vi "Control.vi"() -> ()   [LabVIEW 2023, in "BigSkyControl.lvlib"]
uses:
  BigSkyControl.lvlib
  VISAGlobal.vi
panel:
  out "Temperature(C)":dbl=40.0
  in  "Flashlamp mode":bool
  out "Response History":string="Voltage m0725 V\r\ntemp. CG 40 d  \r\nfire ext       \r\n\rtemp. CG 40 d  \r\nfire ext       \rtemp. CG 40 d  \r\nVoltage m0725 V\r\nLP synch :  1  \r\nstandby        \r\n"
  in  "Command (no > or \\r\\n)":string
  in  "Send Command":bool
  in  "Frequency[Hz]":dbl=10.0 min=0.01 max=56.0 step=0.01 format="%.2g"
  in  "Query Frequency":bool
  in  "Set Frequency":bool
  in  "Query Shutter":bool
  in  "Single QSwitch":bool
  in  "Stop QSwitch":bool
  in  "Start QSwitch":bool
  in  "Query Voltage":bool
  in  "Set Voltage":bool
  in  "Stop":bool
  out "Voltage Reported":dbl=725.0 format="%_4f"
  in  "Voltage[V]":dbl(slide)=725.0 min=700.0 max=950.0 step=5.0 scale=700.0..950.0
  in  "Stop Lamps":bool
  in  "Warmup Lamps":bool
  out "Response":string="Voltage m0725 V\r\n"
  in  "Close shutter":bool
  in  "Open shutter":bool
  in  "VISA resource name":refnum<visa-resource-name>="COM16"
  # "BigSky Laser Control Panel"
  # "System"
  # "Lamp Control"
  # "Q-Switch Control - WILL FIRE LASER"
  # "Shutter Control"
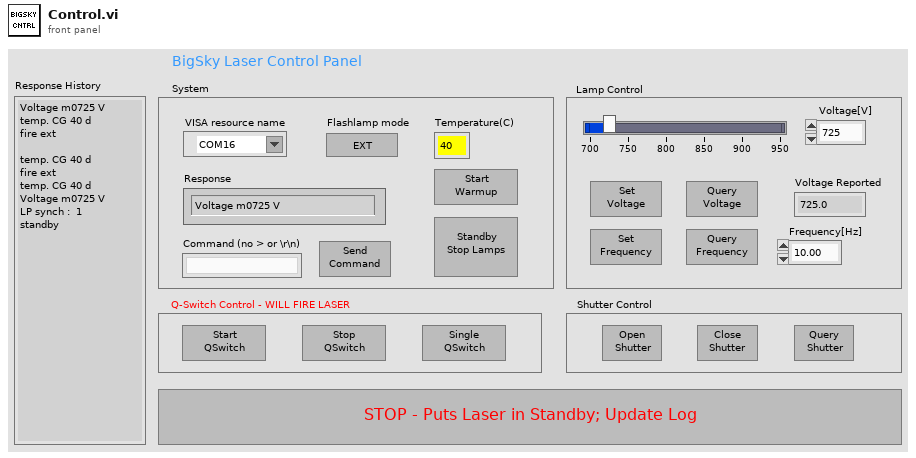
[diagram p1: front panel]
types:
  T1 = enum8{"Enabled", "Disabled", "Disabled and Grayed Out"}
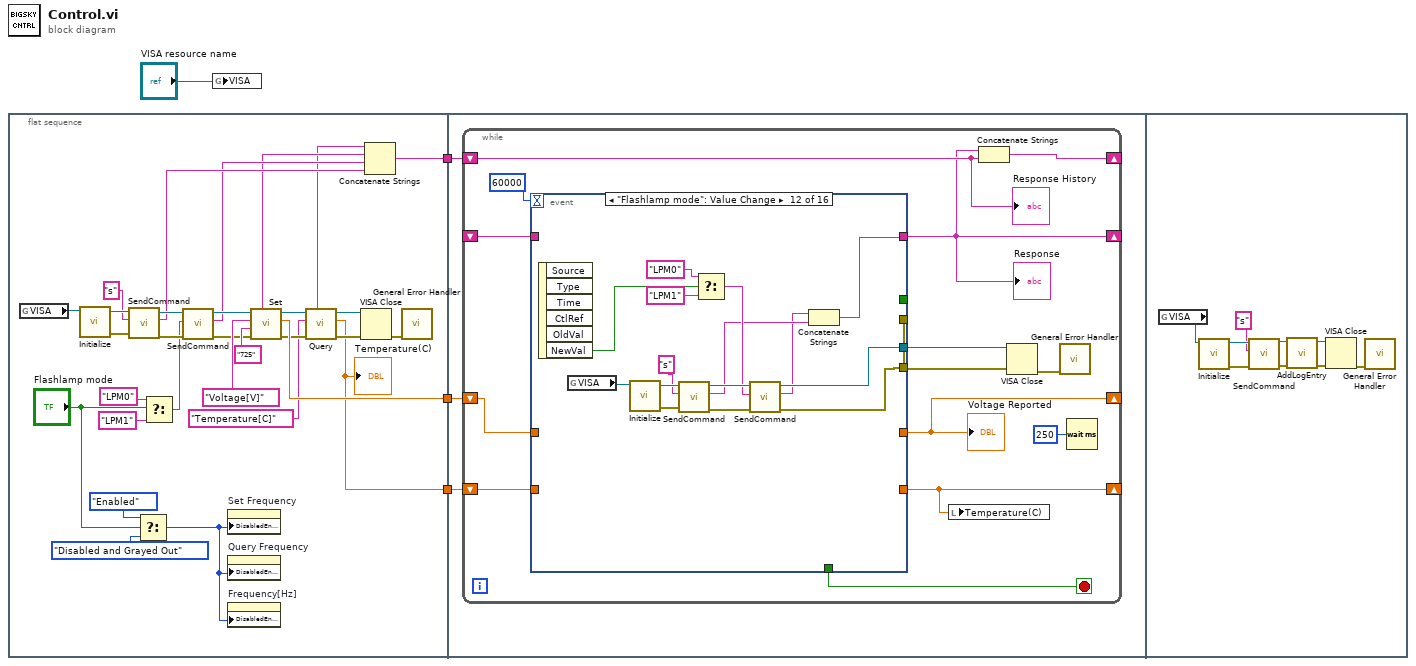
[diagram p0: block diagram]
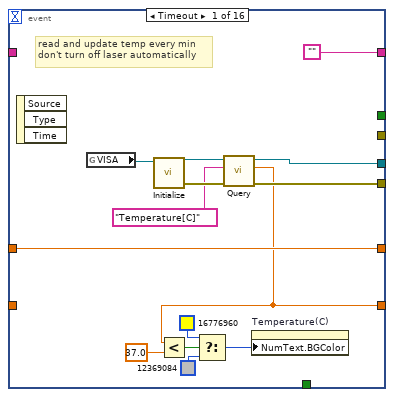
[diagram p2: hidden frame]
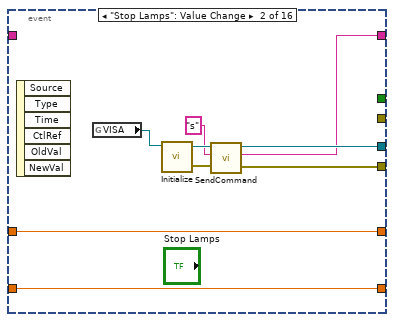
[diagram p3: hidden frame]
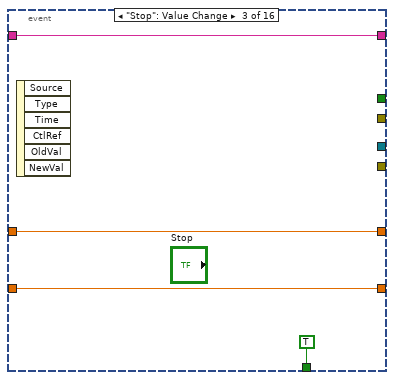
[diagram p4: hidden frame]
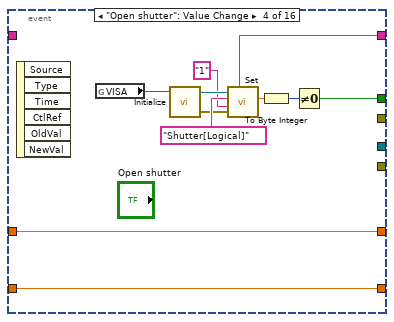
[diagram p5: hidden frame]
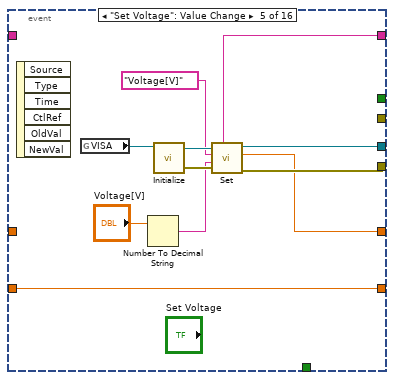
[diagram p6: hidden frame]
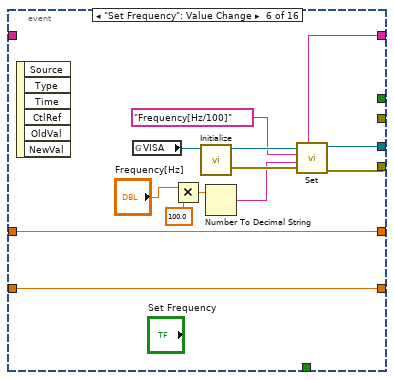
[diagram p7: hidden frame]
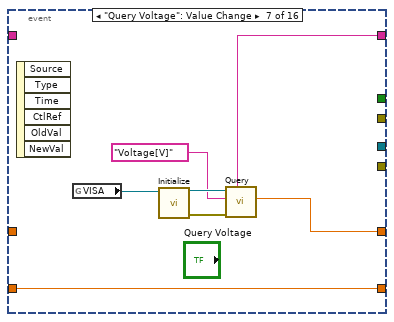
[diagram p8: hidden frame]
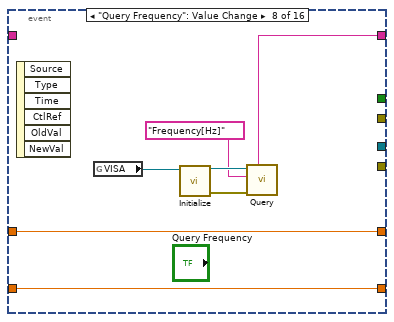
[diagram p9: hidden frame]
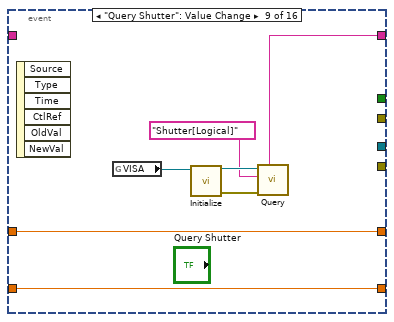
[diagram p10: hidden frame]
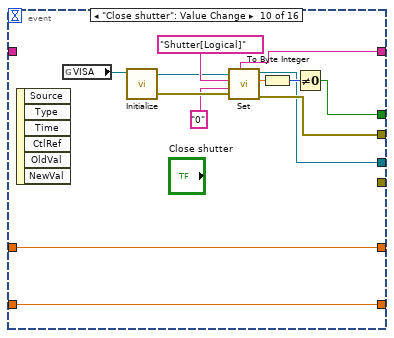
[diagram p11: hidden frame]
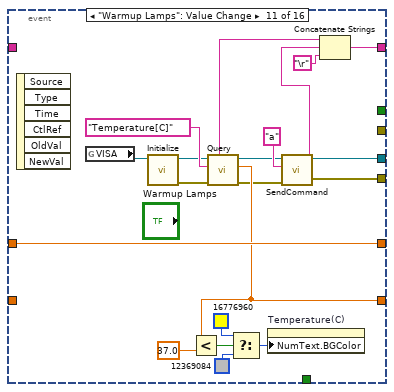
[diagram p12: hidden frame]
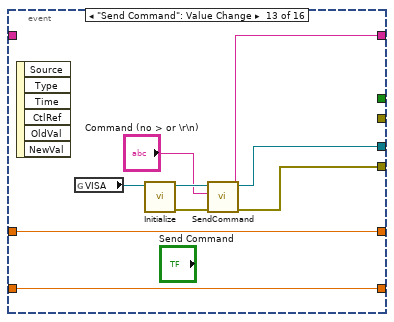
[diagram p13: hidden frame]
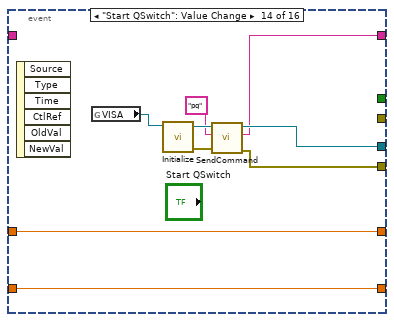
[diagram p14: hidden frame]
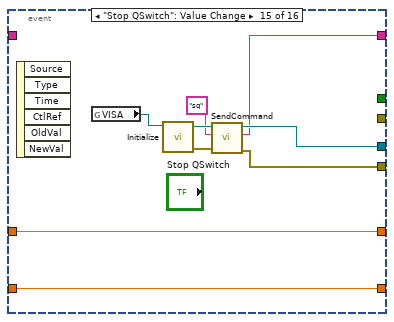
[diagram p15: hidden frame]
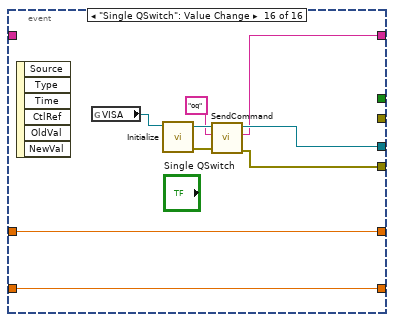
[diagram p16: hidden frame]
diagram:
  n1 = flat-sequence {
    tunnel: [w27] -> w3
    tunnel: [w20] -> w2
    tunnel: [w5] -> w1
    tunnel: w3 -> [w37]
    tunnel: w2 -> [w36]
    tunnel: w1 -> [w35]
    frame #0 {
      n2 = global read "VISAGlobal.vi" "VISA"() -> (w31:refnum<visa-resource-name>)
      n3 = call "Initialize.vi"("VISA resource name"=w31) -> ("error out"=w33:errorcluster, "VISA resource name out"=w34:refnum<visa-resource-name>)  [unwired: 7 in]
      n4 = call "SendCommand.vi"("error"=w33, "write buffer (don't include >\\r\\n)"="s" ("write buffer (don't include >\\r\\n)"), "VISA resource name"=w34) -> ("error out"=w24:errorcluster, "Response"=w9:string, "VISA resource name out"=w26:refnum<visa-resource-name>)  [unwired: 6 in]
      n5 = Select(t=T1."Enabled" ("Disabled"), s="Flashlamp mode", f=T1."Disabled and Grayed Out" ("Disabled")) -> (s? t:f=w10:T1)
      n6 = Select(t="LPM0" ("write buffer (don't include >\\r\\n)"), s="Flashlamp mode", f="LPM1" ("write buffer (don't include >\\r\\n)")) -> (s? t:f=w22:string)
      n7 = call "SendCommand.vi"("error"=w24, "write buffer (don't include >\\r\\n)"=w22, "VISA resource name"=w26) -> ("error out"=w23:errorcluster, "Response"=w8:string, "VISA resource name out"=w25:refnum<visa-resource-name>)  [unwired: 6 in]
      n8 = property on="Set Frequency" class="Bool"("DisabledEnum"=w10) -> ()  [unwired: 2 in, 2 out]
      n9 = property on="Query Frequency" class="Bool"("DisabledEnum"=w10) -> ()  [unwired: 2 in, 2 out]
      n10 = property on="Frequency[Hz]" class="DigNum (strict)"("DisabledEnum"=w10) -> ()  [unwired: 2 in, 2 out]
      n11 = call "Set.vi"("error"=w23, "Input Command String"="725", "Quantity"="Voltage[V]", "VISA resource name"=w25) -> ("error out"=w17:errorcluster, "Returned"=w20:dbl, "VISA resource name out"=w19:refnum<visa-resource-name>, "Response"=w7:string)  [unwired: 2 in]
      n12 = call "Query.vi"("error"=w17, "Quantity"="Temperature[C]", "VISA resource name"=w19) -> ("error out"=w16:errorcluster, "Value"=w5:dbl, "VISA resource name out"=w18:refnum<visa-resource-name>, "Response"=w6:string)  [unwired: 3 in]
      "Temperature(C)" <- w5
      n13 = VISA Close(VISA resource name=w18, error in (no error)=w16) -> (error out=w30:errorcluster)
      n14 = Concatenate Strings(w6, w7, w8, w9) -> (w27:string)
      n15 = call <vilib>:"General Error Handler.vi"("error in (no error)"=w30) -> ()  [unwired: 10 in, 5 out]
    }
    frame #1 {
      n16 = while {
        shift-right: [w40] -> _
        shift-left: _ -> [w45]
        shift-right: [w44] -> _
        shift-left: w36 -> [w43]
        shift-right: [w42] -> _
        shift-left: w37 -> [w41]
        shift-right: [w38] -> _
        shift-left: w35 -> [w39]
        stop <- w47 stop-if-true
        n17 = event shown="[11] \"Flashlamp mode\": Value Change" {
          selector: _ -> [_ _ _ _ _ _ _ _ _ _ _ _ _ _ _ _]
          dyn-events: _ -> [_ _ _ _ _ _ _ _ _ _ _ _ _ _ _ _]
          timeout: 60000 -> [_ _ _ _ _ _ _ _ _ _ _ _ _ _ _ _]
          tunnel: ["" w68 w77 w86 w97 w110 w115 w123 w130 w144 w157 w172 w186 w194 w203 w212] -> w40
          tunnel: [_ _ _ w83 _ _ _ _ _ w141 _ _ _ _ _ _] -> _
          tunnel: [_ _ _ _ _ _ _ _ _ w139 _ _ _ _ _ _] -> w51
          tunnel: [w64 w70 _ _ w93 w108 _ _ _ w138 w151 w171 w188 w195 w204 w213] -> w50
          tunnel: [w63 w69 _ _ w92 w107 _ _ _ _ w148 w170 w187 w196 w205 w214] -> _
          tunnel: [_ _ TRUE _ _ _ _ _ _ _ _ _ _ _ _ _] -> w47
          tunnel: [w65 w67 w76 w80 w91 w101 w116 w122 w129 w136 w165 _ w185 w192 w202 w211] -> w44
          tunnel: w45 -> [_ _ w77 _ _ _ _ _ _ _ _ _ _ _ _ _]
          tunnel: w43 -> [w65 w67 w76 w80 _ w101 _ w122 w129 w136 w165 _ w185 w192 w202 w211]
          tunnel: w39 -> [_ w66 w75 w79 w90 w102 w114 w121 w128 w135 _ _ w183 w193 w201 w210]
          tunnel: [w58 w66 w75 w79 w90 w102 w114 w121 w128 w135 w162 _ w183 w193 w201 w210] -> w38
          event Timeout {
            # "read and update temp every min\ndon't turn off laser automatically"
            n18 = event-data() -> ()  [unwired: 1 in, 3 out]
            n19 = global read "VISAGlobal.vi" "VISA"() -> (w60:refnum<visa-resource-name>)
            n20 = call "Initialize.vi"("VISA resource name"=w60) -> ("error out"=w61:errorcluster, "VISA resource name out"=w62:refnum<visa-resource-name>)  [unwired: 7 in]
            n21 = call "Query.vi"("error"=w61, "Quantity"="Temperature[C]", "VISA resource name"=w62) -> ("error out"=w63:errorcluster, "Value"=w58:dbl, "VISA resource name out"=w64:refnum<visa-resource-name>)  [unwired: 3 in, 1 out]
            n22 = Less?(x=w58, y=37.0) -> (x < y?=w54:bool)
            n23 = Select(t=u32 16776960 ("Color"), s=w54, f=u32 12369084 ("Color")) -> (s? t:f=w53:u32)
            n24 = property on="Temperature(C)" class="DigNum (strict)"("NumText.BGColor"=w53) -> ()  [unwired: 2 in, 2 out]
          }
          event "Stop Lamps": Value Change {
            n25 = event-data() -> ()  [unwired: 1 in, 6 out]
            n26 = global read "VISAGlobal.vi" "VISA"() -> (w71:refnum<visa-resource-name>)
            n27 = call "Initialize.vi"("VISA resource name"=w71) -> ("error out"=w73:errorcluster, "VISA resource name out"=w74:refnum<visa-resource-name>)  [unwired: 7 in]
            n28 = call "SendCommand.vi"("error"=w73, "write buffer (don't include >\\r\\n)"="s" ("write buffer (don't include >\\r\\n)"), "VISA resource name"=w74) -> ("error out"=w69:errorcluster, "Response"=w68:string, "VISA resource name out"=w70:refnum<visa-resource-name>)  [unwired: 6 in]
          }
          event "Stop": Value Change {
            n29 = event-data() -> ()  [unwired: 1 in, 6 out]
          }
          event "Open shutter": Value Change {
            n30 = event-data() -> ()  [unwired: 1 in, 6 out]
            n31 = global read "VISAGlobal.vi" "VISA"() -> (w81:refnum<visa-resource-name>)
            n32 = call "Initialize.vi"("VISA resource name"=w81) -> ("error out"=w87:errorcluster, "VISA resource name out"=w88:refnum<visa-resource-name>)  [unwired: 7 in]
            n33 = call "Set.vi"("error"=w87, "Input Command String"="1", "Quantity"="Shutter[Logical]", "VISA resource name"=w88) -> ("Returned"=w85:dbl, "Response"=w86:string)  [unwired: 2 in, 2 out]
            n34 = To Byte Integer(number=w85) -> (8bit integer=w84:i8)
            n35 = Not Equal To 0?(x=w84) -> (x != 0?=w83:bool)
          }
          event "Set Voltage": Value Change {
            n36 = event-data() -> ()  [unwired: 1 in, 6 out]
            n37 = global read "VISAGlobal.vi" "VISA"() -> (w98:refnum<visa-resource-name>)
            n38 = Number To Decimal String(number="Voltage[V]") -> (decimal integer string=w94:string)  [unwired: 1 in]
            n39 = call "Initialize.vi"("VISA resource name"=w98) -> ("error out"=w99:errorcluster, "VISA resource name out"=w100:refnum<visa-resource-name>)  [unwired: 7 in]
            n40 = call "Set.vi"("error"=w99, "Input Command String"=w94, "Quantity"="Voltage[V]", "VISA resource name"=w100) -> ("error out"=w92:errorcluster, "Returned"=w91:dbl, "VISA resource name out"=w93:refnum<visa-resource-name>, "Response"=w97:string)  [unwired: 2 in]
          }
          event "Set Frequency": Value Change {
            n41 = event-data() -> ()  [unwired: 1 in, 6 out]
            n42 = global read "VISAGlobal.vi" "VISA"() -> (w111:refnum<visa-resource-name>)
            n43 = Multiply(x="Frequency[Hz]", y=100.0) -> (x*y=w104:dbl)
            n44 = call "Initialize.vi"("VISA resource name"=w111) -> ("error out"=w112:errorcluster, "VISA resource name out"=w113:refnum<visa-resource-name>)  [unwired: 7 in]
            n45 = Number To Decimal String(number=w104) -> (decimal integer string=w109:string)  [unwired: 1 in]
            n46 = call "Set.vi"("error"=w112, "Input Command String"=w109, "Quantity"="Frequency[Hz/100]", "VISA resource name"=w113) -> ("error out"=w107:errorcluster, "VISA resource name out"=w108:refnum<visa-resource-name>, "Response"=w110:string)  [unwired: 2 in, 1 out]
          }
          event "Query Voltage": Value Change {
            n47 = event-data() -> ()  [unwired: 1 in, 6 out]
            n48 = global read "VISAGlobal.vi" "VISA"() -> (w118:refnum<visa-resource-name>)
            n49 = call "Initialize.vi"("VISA resource name"=w118) -> ("error out"=w119:errorcluster, "VISA resource name out"=w120:refnum<visa-resource-name>)  [unwired: 7 in]
            n50 = call "Query.vi"("error"=w119, "Quantity"="Voltage[V]", "VISA resource name"=w120) -> ("Value"=w116:dbl, "Response"=w115:string)  [unwired: 3 in, 2 out]
          }
          event "Query Frequency": Value Change {
            n51 = event-data() -> ()  [unwired: 1 in, 6 out]
            n52 = global read "VISAGlobal.vi" "VISA"() -> (w125:refnum<visa-resource-name>)
            n53 = call "Initialize.vi"("VISA resource name"=w125) -> ("error out"=w126:errorcluster, "VISA resource name out"=w127:refnum<visa-resource-name>)  [unwired: 7 in]
            n54 = call "Query.vi"("error"=w126, "Quantity"="Frequency[Hz]", "VISA resource name"=w127) -> ("Response"=w123:string)  [unwired: 3 in, 3 out]
          }
          event "Query Shutter": Value Change {
            n55 = event-data() -> ()  [unwired: 1 in, 6 out]
            n56 = global read "VISAGlobal.vi" "VISA"() -> (w132:refnum<visa-resource-name>)
            n57 = call "Initialize.vi"("VISA resource name"=w132) -> ("error out"=w133:errorcluster, "VISA resource name out"=w134:refnum<visa-resource-name>)  [unwired: 7 in]
            n58 = call "Query.vi"("error"=w133, "Quantity"="Shutter[Logical]", "VISA resource name"=w134) -> ("Response"=w130:string)  [unwired: 3 in, 3 out]
          }
          event "Close shutter": Value Change {
            n59 = event-data() -> ()  [unwired: 1 in, 6 out]
            n60 = global read "VISAGlobal.vi" "VISA"() -> (w137:refnum<visa-resource-name>)
            n61 = call "Initialize.vi"("VISA resource name"=w137) -> ("error out"=w145:errorcluster, "VISA resource name out"=w146:refnum<visa-resource-name>)  [unwired: 7 in]
            n62 = call "Set.vi"("error"=w145, "Input Command String"="0", "Quantity"="Shutter[Logical]", "VISA resource name"=w146) -> ("error out"=w139:errorcluster, "Returned"=w143:dbl, "VISA resource name out"=w138:refnum<visa-resource-name>, "Response"=w144:string)  [unwired: 2 in]
            n63 = To Byte Integer(number=w143) -> (8bit integer=w142:i8)
            n64 = Not Equal To 0?(x=w142) -> (x != 0?=w141:bool)
          }
          event "Warmup Lamps": Value Change {
            n65 = event-data() -> ()  [unwired: 1 in, 6 out]
            n66 = global read "VISAGlobal.vi" "VISA"() -> (w166:refnum<visa-resource-name>)
            n67 = call "Initialize.vi"("VISA resource name"=w166) -> ("error out"=w150:errorcluster, "VISA resource name out"=w153:refnum<visa-resource-name>)  [unwired: 7 in]
            n68 = call "Query.vi"("error"=w150, "Quantity"="Temperature[C]", "VISA resource name"=w153) -> ("error out"=w149:errorcluster, "Value"=w162:dbl, "VISA resource name out"=w152:refnum<visa-resource-name>, "Response"=w156:string)  [unwired: 3 in]
            n69 = Less?(x=w162, y=37.0) -> (x < y?=w161:bool)
            n70 = Select(t=u32 16776960 ("Color"), s=w161, f=u32 12369084 ("Color")) -> (s? t:f=w160:u32)
            n71 = property on="Temperature(C)" class="DigNum (strict)"("NumText.BGColor"=w160) -> ()  [unwired: 2 in, 2 out]
            n72 = call "SendCommand.vi"("error"=w149, "write buffer (don't include >\\r\\n)"="a" ("write buffer (don't include >\\r\\n)"), "VISA resource name"=w152) -> ("error out"=w148:errorcluster, "Response"=w155:string, "VISA resource name out"=w151:refnum<visa-resource-name>)  [unwired: 6 in]
            n73 = Concatenate Strings(w156, w155, "\r") -> (w157:string)
          }
          event "Flashlamp mode": Value Change {
            n74 = event-data() -> ("NewVal"=w174:bool)  [unwired: 1 in, 5 out]
            n75 = global read "VISAGlobal.vi" "VISA"() -> (w180:refnum<visa-resource-name>)
            n76 = call "Initialize.vi"("VISA resource name"=w180) -> ("error out"=w181:errorcluster, "VISA resource name out"=w182:refnum<visa-resource-name>)  [unwired: 7 in]
            n77 = call "SendCommand.vi"("error"=w181, "write buffer (don't include >\\r\\n)"="s" ("write buffer (don't include >\\r\\n)"), "VISA resource name"=w182) -> ("error out"=w178:errorcluster, "Response"=w169:string, "VISA resource name out"=w177:refnum<visa-resource-name>)  [unwired: 6 in]
            n78 = Select(t="LPM0" ("write buffer (don't include >\\r\\n)"), s=w174, f="LPM1" ("write buffer (don't include >\\r\\n)")) -> (s? t:f=w173:string)
            n79 = call "SendCommand.vi"("error"=w178, "write buffer (don't include >\\r\\n)"=w173, "VISA resource name"=w177) -> ("error out"=w170:errorcluster, "Response"=w168:string, "VISA resource name out"=w171:refnum<visa-resource-name>)  [unwired: 6 in]
            n80 = Concatenate Strings(w168, w169) -> (w172:string)
          }
          event "Send Command": Value Change {
            n81 = event-data() -> ()  [unwired: 1 in, 6 out]
            n82 = global read "VISAGlobal.vi" "VISA"() -> (w189:refnum<visa-resource-name>)
            n83 = call "Initialize.vi"("VISA resource name"=w189) -> ("error out"=w190:errorcluster, "VISA resource name out"=w191:refnum<visa-resource-name>)  [unwired: 7 in]
            n84 = call "SendCommand.vi"("error"=w190, "write buffer (don't include >\\r\\n)"="Command (no > or \\r\\n)", "VISA resource name"=w191) -> ("error out"=w187:errorcluster, "Response"=w186:string, "VISA resource name out"=w188:refnum<visa-resource-name>)  [unwired: 6 in]
          }
          event "Start QSwitch": Value Change {
            n85 = event-data() -> ()  [unwired: 1 in, 6 out]
            n86 = global read "VISAGlobal.vi" "VISA"() -> (w197:refnum<visa-resource-name>)
            n87 = call "Initialize.vi"("VISA resource name"=w197) -> ("error out"=w199:errorcluster, "VISA resource name out"=w200:refnum<visa-resource-name>)  [unwired: 7 in]
            n88 = call "SendCommand.vi"("error"=w199, "write buffer (don't include >\\r\\n)"="pq" ("write buffer (don't include >\\r\\n)"), "VISA resource name"=w200) -> ("error out"=w196:errorcluster, "Response"=w194:string, "VISA resource name out"=w195:refnum<visa-resource-name>)  [unwired: 6 in]
          }
          event "Stop QSwitch": Value Change {
            n89 = event-data() -> ()  [unwired: 1 in, 6 out]
            n90 = global read "VISAGlobal.vi" "VISA"() -> (w206:refnum<visa-resource-name>)
            n91 = call "Initialize.vi"("VISA resource name"=w206) -> ("error out"=w208:errorcluster, "VISA resource name out"=w209:refnum<visa-resource-name>)  [unwired: 7 in]
            n92 = call "SendCommand.vi"("error"=w208, "write buffer (don't include >\\r\\n)"="sq" ("write buffer (don't include >\\r\\n)"), "VISA resource name"=w209) -> ("error out"=w205:errorcluster, "Response"=w203:string, "VISA resource name out"=w204:refnum<visa-resource-name>)  [unwired: 6 in]
          }
          event "Single QSwitch": Value Change {
            n93 = event-data() -> ()  [unwired: 1 in, 6 out]
            n94 = global read "VISAGlobal.vi" "VISA"() -> (w215:refnum<visa-resource-name>)
            n95 = call "Initialize.vi"("VISA resource name"=w215) -> ("error out"=w217:errorcluster, "VISA resource name out"=w218:refnum<visa-resource-name>)  [unwired: 7 in]
            n96 = call "SendCommand.vi"("error"=w217, "write buffer (don't include >\\r\\n)"="oq" ("write buffer (don't include >\\r\\n)"), "VISA resource name"=w218) -> ("error out"=w214:errorcluster, "Response"=w212:string, "VISA resource name out"=w213:refnum<visa-resource-name>)  [unwired: 6 in]
          }
        }
        "Response" <- w40
        "Voltage Reported" <- w44
        n97 = local write "Temperature(C)"(w38) -> ()
        n98 = Concatenate Strings(w40, w41) -> (w42:string)
        n99 = VISA Close(VISA resource name=w50, error in (no error)=w51) -> (error out=w49:errorcluster)
        n100 = call <vilib>:"General Error Handler.vi"("error in (no error)"=w49) -> ()  [unwired: 10 in, 5 out]
        n101 = Wait (ms)(milliseconds to wait=u32 250) -> ()  [unwired: 1 out]
        "Response History" <- w41
      }
    }
    frame #2 {
      n102 = global read "VISAGlobal.vi" "VISA"() -> (w224:refnum<visa-resource-name>)
      n103 = call "Initialize.vi"("VISA resource name"=w224) -> ("error out"=w226:errorcluster, "VISA resource name out"=w227:refnum<visa-resource-name>)  [unwired: 7 in]
      n104 = call "SendCommand.vi"("error"=w226, "write buffer (don't include >\\r\\n)"="s" ("write buffer (don't include >\\r\\n)"), "VISA resource name"=w227) -> ("error out"=w220:errorcluster, "VISA resource name out"=w222:refnum<visa-resource-name>)  [unwired: 6 in, 1 out]
      n105 = call "AddLogEntry.vi"("error in (no error)"=w220, "VISA Refnum in"=w222) -> ("error out"=w219:errorcluster, "VISA Refnum out"=w221:refnum<visa-resource-name>)  [unwired: 8 in]
      n106 = VISA Close(VISA resource name=w221, error in (no error)=w219) -> (error out=w223:errorcluster)
      n107 = call <vilib>:"General Error Handler.vi"("error in (no error)"=w223) -> ()  [unwired: 10 in, 5 out]
    }
  }
  n108 = global write "VISAGlobal.vi" "VISA"("VISA resource name") -> ()
